vi "RichToFlatrouteguide_Point.vi"(5 "OutputClusterType":T1, 11 "InputCluster":T2) -> (3 "OutputCluster":T1)   [LabVIEW 2019, in "Generated_server.lvlib"]
uses:
  Generated_server.lvlib
  routeguide_Point.ctl
  routeguide_Point_Flat.ctl
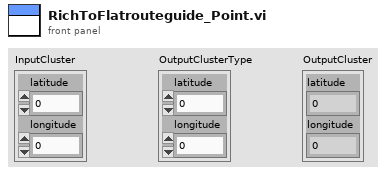
[diagram p1: front panel]
types:
  T1 = typedef "Generated_server.lvlib/routeguide_Point_Flat.ctl" = cluster{"latitude":i32, "longitude":i32}
  T2 = typedef "Generated_server.lvlib/routeguide_Point.ctl" = cluster{"latitude":i32, "longitude":i32}
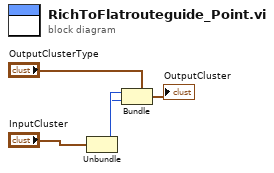
[diagram p0: block diagram]
diagram:
  n1 = Unbundle "Unbundle"("InputCluster") -> ("latitude"=w2:i32, "longitude"=w1:i32)
  n2 = Bundle "Bundle"(cluster="OutputClusterType", "latitude"=w2, "longitude"=w1) -> (→"OutputCluster":T1)
